vi "Read Frame_Data.vi"(8 "error in (no error)":errorcluster, 11 "Config_Read in":refnum<class "Config_Read_BML.lvclass">) -> (0 "error out":errorcluster, 2 "FRM_Data_Array":T1[](array[typedef]) {"Data" format="%x"; "Start_Addr" format="%x"}, 3 "Config_Read out":refnum<class "Config_Read_BML.lvclass">)   [LabVIEW 2018, in "Config_Read_BML.lvclass"]
uses:
  Config_Read_BML.lvclass
  Frame_Data.ctl
  OperationMode.ctl
  BurstLength.ctl
  RW_Option.ctl
  Config_Read_BML.lvclass/Config_Read_BML.ctl
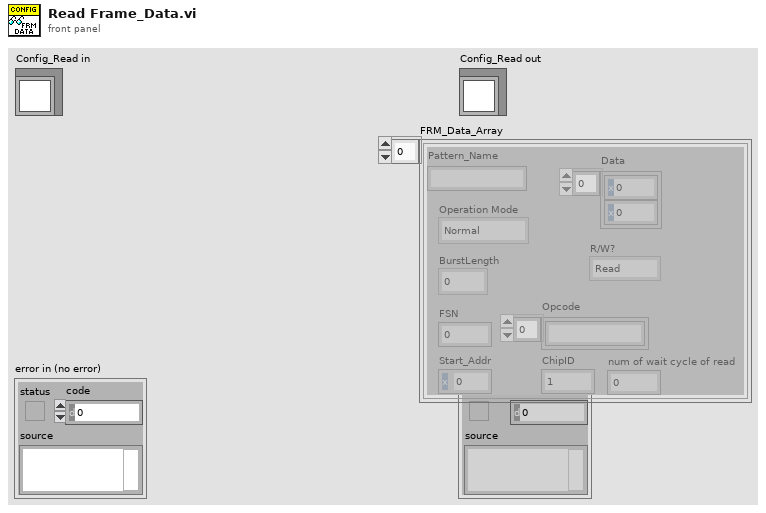
[diagram p1: front panel]
types:
  T1 = typedef "Config_Read_BML.lvclass/Frame_Data.ctl" = cluster{"Pattern_Name":string, "Operation Mode":T2, "BurstLength":T3, "FSN":u8, "Start_Addr":u16, "Data":u8[], "R/W?":T4, "Opcode":string[], "ChipID":u8, "num of wait cycle of read":i8}
  T2 = typedef "Config_Read_BML.lvclass/OperationMode.ctl" = enum8{"Normal", "ImmeEffect", "InitSlaveID", "LoadData"}
  T3 = typedef "Config_Read_BML.lvclass/BurstLength.ctl" = enum8{"0", "2", "3", "4", "5", "8", "16", "32"}
  T4 = typedef "Config_Read_BML.lvclass/RW_Option.ctl" = enum16{"Read", "Write", "R/W"}
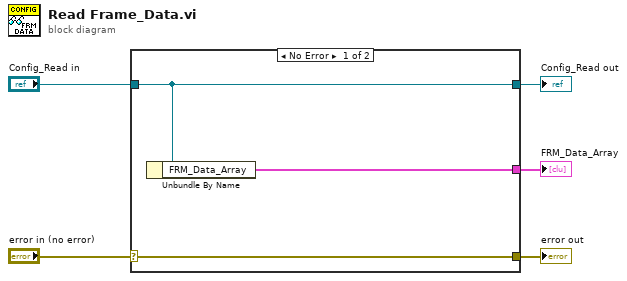
[diagram p0: block diagram]
diagram:
  n1 = case shown="No Error" "error in (no error)" {
    selector: "error in (no error)" -> [w8 w9]
    tunnel: [w8 w9] -> w4
    tunnel: [w7 w10] -> w2
    tunnel: "Config_Read in" -> [w7 w10]
    tunnel: [w6 _] -> w1
    frame No Error {
      n2 = Unbundle By Name(w7) -> ("FRM_Data_Array"=w6:T1[])
    }
    frame Error {
    }
  }
  "error out" <- w4
  "Config_Read out" <- w2
  "FRM_Data_Array" <- w1
